vi "Insight_RW_Laser_ON-OFF_mode.vi"(7 "Command Version":enum8{":CONF:SWE:CONT", ":SYSTem:CONTrol"}(ring), 8 "error in (no error)":errorcluster, 9 "Mode (Read / Write)":enum8{"Write", "Read"}(ring), 10 "Laser ON Mode":enum8{"Hardware", "Software"}(ring)=enum."Software", 11 "telnet connection":T1) -> (0 "error out":errorcluster, 1 "full response data":string, 2 "Laser ON Mode":enum8{"Hardware", "Software"}(ring)=enum."Software", 3 "telnet connection out":T1)   [LabVIEW 2011]
doc: "Insight Photonic Solutions\n\nThis VI reads or writes the control parameter for how the Laser outputs light: via Hardware or Software control. The control value may be 1 = Hardware mode, or 2 = Software mode.\n\nIn Hardware mode, the Laser ON switch or a GPIO digital line control when light is emitted from the laser and a sweep is started or stopped.\n\nIn Software mode, :INIT:SWEep starts sweeps and emits light from the laser, and :ABORt cancels sweeps extiniguishes light from the laser. The Laser ON switch state, and the GPIO line, are ignored.\n\nAfter Atlas v2.2.0, the command syntax changed. We added an input to select the correct syntax depending on the Atlas code version:\n\nversion 2.2.0 or older, command is :CONFigure:SWEep:CONTrol\nafter v2.2.0, command is :SYSTem:CONTrol\n\nver 1.0 - original release\nver 2.0 - capture errors from invalid command; add enum selector for old and new versions of this command\nver 3.2 - handle parser responses from Atlas 3.2 and later, or version 3.1 and earlier."
uses:
  Telnet Session.ctl
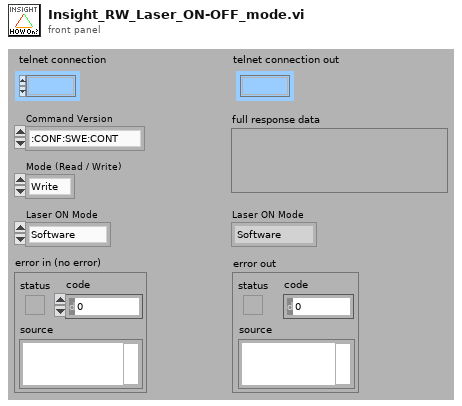
[diagram p1: front panel]
types:
  T1 = typedef "Telnet Session.ctl" = refnum<k1>
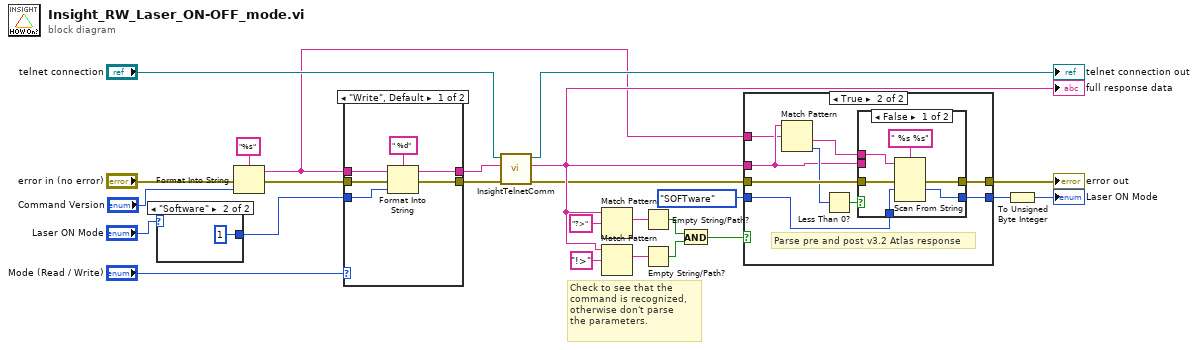
[diagram p0: block diagram]
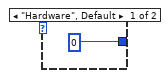
[diagram p2: hidden frame]
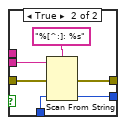
[diagram p4: hidden frame]
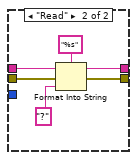
[diagram p5: hidden frame]
diagram:
  # "Check to see that the \ncommand is recognized,\notherwise don't parse \nthe parameters."
  n1 = case shown="\"Software\"" "Laser ON Mode" {
    tunnel: [u8 0 u8 1] -> w1
    frame "Hardware", Default {
    }
    frame "Software" {
    }
  }
  n2 = Format Into String(format string="%s", error in="error in (no error)", "Command Version") -> (resulting string=w6:string, error out=w8:errorcluster)  [unwired: 1 in]
  n3 = case shown="\"Write\", Default" "Mode (Read / Write)" {
    tunnel: [w33 w37] -> w24
    tunnel: w8 -> [w32 w36]
    tunnel: w1 -> [w29 _]
    tunnel: [w30 w38] -> w23
    tunnel: w6 -> [w28 w35]
    frame "Write", Default {
      n4 = Format Into String(format string=" %d", initial string=w28, error in=w32, w29) -> (resulting string=w30:string, error out=w33:errorcluster)
    }
    frame "Read" {
      n5 = Format Into String(format string="%s", initial string=w35, error in=w36, "?" ("input 1")) -> (resulting string=w38:string, error out=w37:errorcluster)
    }
  }
  n6 = call "InsightTelnetComm.vi"("error in"=w24, "write buffer (\"\")"=w23, "telnet connection"="telnet connection") -> ("error out"=w13:errorcluster, "response data"=w14:string, "telnet  connection out"=→"telnet connection out":T1)  [unwired: 4 in]
  "full response data" <- w14
  n7 = Match Pattern(string=w14, regular expression="?>") -> (match substring=w16:string)  [unwired: 1 in, 3 out]
  n8 = Match Pattern(string=w14, regular expression="!>") -> (match substring=w17:string)  [unwired: 1 in, 3 out]
  n9 = Empty String/Path?(string/path=w16) -> (empty?=w19:bool)
  n10 = Empty String/Path?(string/path=w17) -> (empty?=w20:bool)
  n11 = And(x=w19, y=w20) -> (x .and. y?=w11:bool)
  n12 = case shown="True" w11 {
    tunnel: [w41 w48] -> w12
    tunnel: w13 -> [w41 w47]
    tunnel: w14 -> [_ w44]
    tunnel: [w40 w49] -> w4
    tunnel: w6 -> [_ w43]
    tunnel: enum16{"HARDware", "SOFTware"}."SOFTware" -> [w40 w42]
    frame False {
    }
    frame True {
      # "Parse pre and post v3.2 Atlas response"
      n13 = Match Pattern(string=w44, regular expression=w43) -> (after substring=w45:string, offset past match=w46:i32)  [unwired: 1 in, 2 out]
      n14 = Less Than 0?(x=w46) -> (x < 0?=w50:bool)
      n15 = case shown="False" w50 {
        tunnel: w45 -> [w55 _]
        tunnel: w44 -> [_ w61]
        tunnel: [w56 w62] -> w48
        tunnel: [w53 w59] -> w49
        tunnel: w47 -> [w52 w58]
        tunnel: w42 -> [w51 w57]
        frame False {
          n16 = Scan From String(format string=" %s %s" ("f"), input string=w55, error in=w52, default 1=w51) -> (error out=w56:errorcluster, output 1=w53:enum16{"HARDware", "SOFTware"})  [unwired: 3 in, 2 out]
        }
        frame True {
          n17 = Scan From String(format string="%[^:]: %s", input string=w61, error in=w58, default 2=w57) -> (error out=w62:errorcluster, output 2=w59:enum16{"HARDware", "SOFTware"})  [unwired: 3 in, 2 out]
        }
      }
    }
  }
  "error out" <- w12
  n18 = To Unsigned Byte Integer(number=w4) -> (unsigned 8bit integer=→"Laser ON Mode":u8)
